vi "Add cell to table Header or Footer.vi"(4 "font":refnum<k24>, 5 "Close Cell ref (T)":bool=TRUE, 6 "Leading":T1=18.0, 7 "Aligment":string="JUSTIFY", 8 "error in (no error)":errorcluster, 9 "Cell format":T2={"Font"={"Name"="Helvetica", "Size"=12.0, "Color"=0, "Style"={"Bold"=FALSE, "Italic"=FALSE, "Underline"=FALSE, "Strikeout"=FALSE}}, "Align. and LS"={"Horizontal"=enum."LEFT", "Vertical"=enum."BOTTOM", "Line spacing"=enum."1.0"}, "Border"={"Show?"=FALSE, "Thickness (point)"=0.0, "Color"=0}}, 10 "String":string, 11 "PdfP Table":refnum<k24>) -> (0 "error out":errorcluster, 2 "Cell ref":refnum<k24>, 3 "PdfP Table duplicate":refnum<k24>)   [LabVIEW 2019]
doc: "Version 1.0\nDeveloped by Jean-Marc Simard\nCopyright © 2010, Exaprom Inc.\nAll rights reserved.\nLicense: BSD\n\nWith iTextSharp 4.1.6 (http://itextsharp.sourceforge.net)\nunder Mozilla Public License Version 1.1\n(http://www.mozilla.org/MPL/MPL-1.1.html)"
uses:
  C:/Program Files/National Instruments/LabVIEW 2019/user.lib/Exaprom PDF/DLL/itextsharp.dll
  DLL/itextsharp.dll
  <userlib>/Exaprom PDF/Controls/Cell Properties.ctl
  <userlib>/Exaprom PDF/Controls/Font Controls/Font cluster.ctl
  <userlib>/Exaprom PDF/Controls/Font Controls/Font size.ctl
  <userlib>/Exaprom PDF/Controls/Font Controls/Font color.ctl
  <userlib>/Exaprom PDF/Controls/Table Controls/Cell Vertical alignment.ctl
  <userlib>/Exaprom PDF/Controls/Text Controls/Line spacing.ctl
  <userlib>/Exaprom PDF/Controls/Image Controls/Image border.ctl
  <userlib>/Exaprom PDF/Controls/Text Controls/Texte alignement.ctl
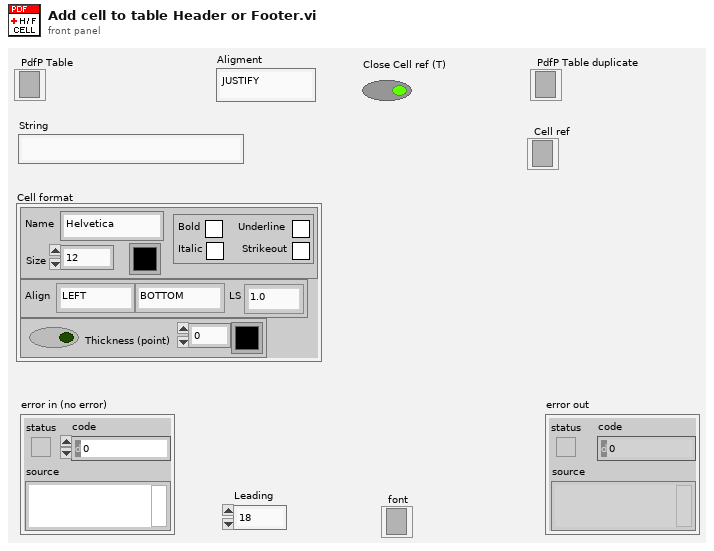
[diagram p1: front panel]
types:
  T1 = typedef "Font size.ctl" = sgl
  T2 = typedef "Cell Properties.ctl" = cluster{"Font":T3, "Align. and LS":cluster{"Horizontal":T5, "Vertical":T6, "Line spacing":T7}, "Border":T8}
  T3 = typedef "Font cluster.ctl" = cluster{"Name":string, "Size":T1, "Color":T4, "Style":cluster{"Bold":bool, "Italic":bool, "Underline":bool, "Strikeout":bool}}
  T4 = typedef "Font color.ctl" = u32
  T5 = typedef "Texte alignement.ctl" = enum16{"Select", "CENTER", "JUSTIFY", "LEFT", "RIGHT"}
  T6 = typedef "Cell Vertical alignment.ctl" = enum16{"TOP", "MIDDLE", "BOTTOM"}
  T7 = typedef "Line spacing.ctl" = enum16{"Select", "1.0", "1.5", "2.0"}
  T8 = typedef "Image border.ctl" = cluster{"Show?":bool, "Thickness (point)":sgl, "Color":u32}
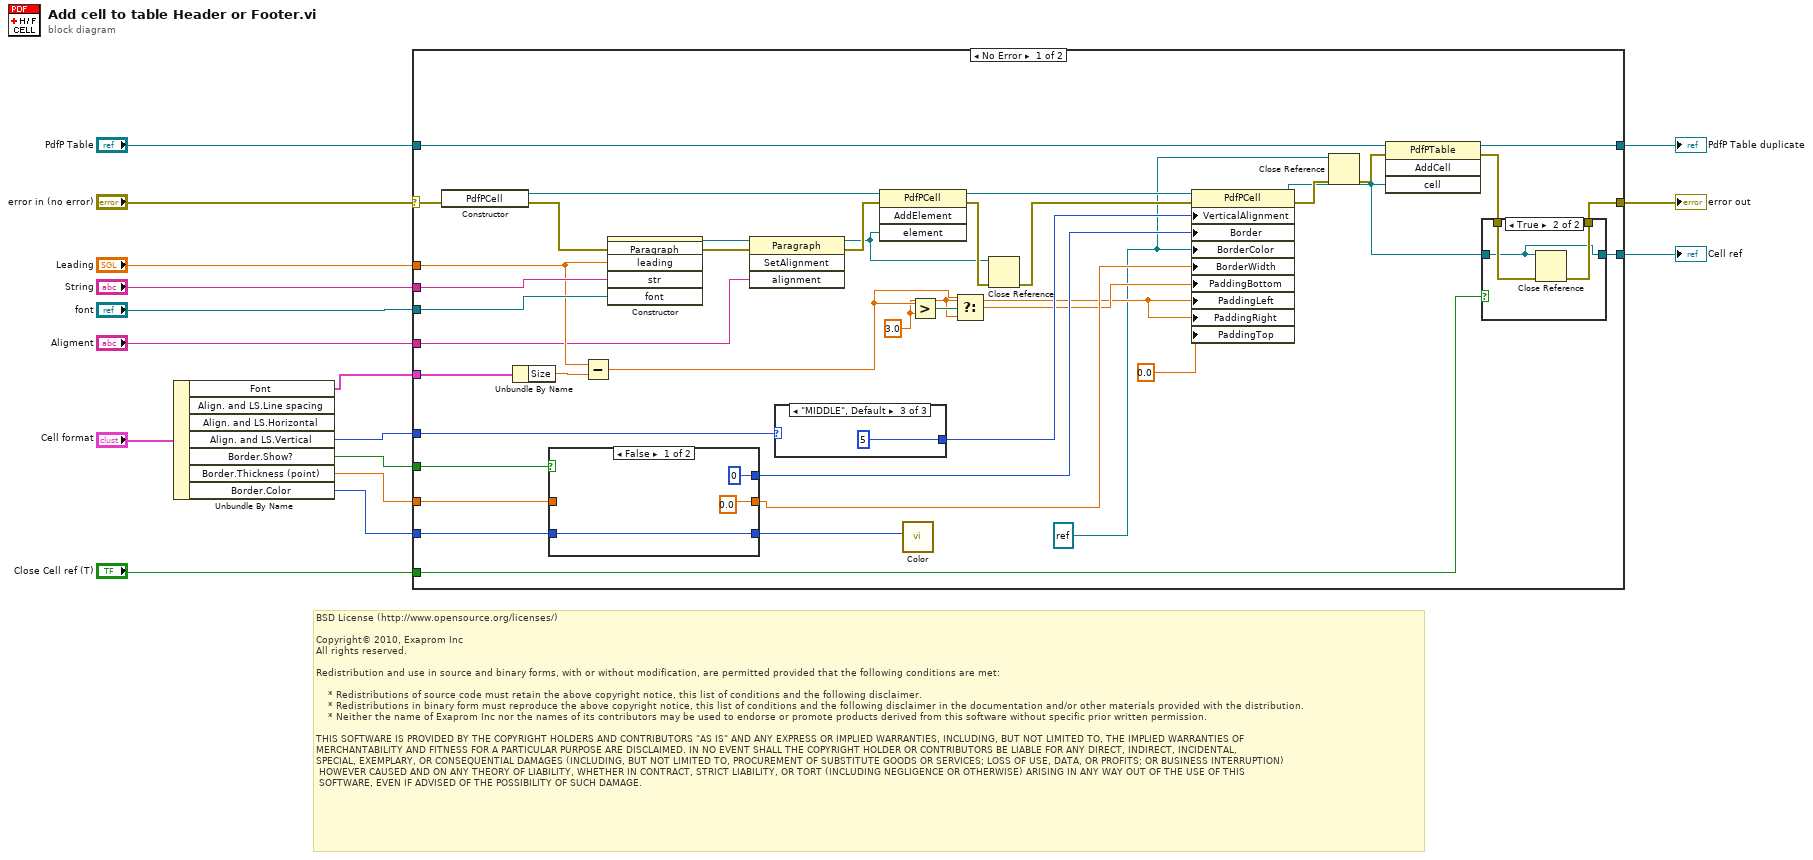
[diagram p0: block diagram]
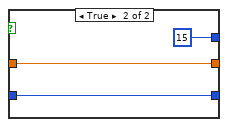
[diagram p3: hidden frame]
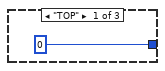
[diagram p4: hidden frame]
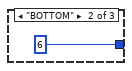
[diagram p5: hidden frame]
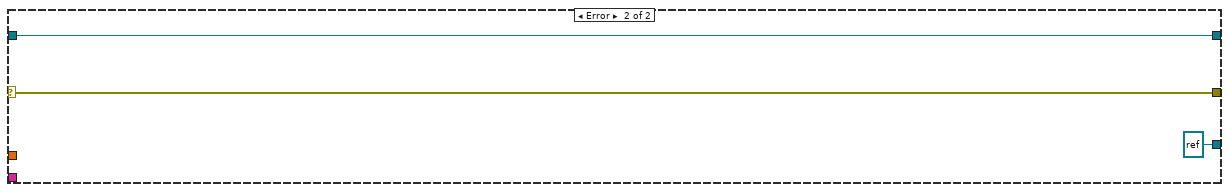
[diagram p6: hidden frame]
diagram:
  # "BSD License (http://www.opensource.org/licenses/)\n\nCopyright© 2010, Exaprom Inc\nAll rights reserved.\n\nRedistribution and use in source and binary forms, with or without modification, are permitted provided that the following conditions are met:\n\n    * Redistributions of source code must retain the above copyright notice, this list of conditions and the following disclaimer.\n    * Redistributions in binary form must reproduce the above copyright notice, this list of conditions and the following disclaimer in the documentation and/or other materials provided with the distribution.\n    * Neither the name of Exaprom Inc nor the names of its contributors may be used to endorse or promote products derived from this software without specific prior written permission.\n\nTHIS SOFTWARE IS PROVIDED BY THE COPYRIGHT HOLDERS AND CONTRIBUTORS \"AS IS\" AND ANY EXPRESS OR IMPLIED WARRANTIES, INCLUDING, BUT NOT LIMITED TO, THE IMPLIED WARRANTIES OF \nMERCHANTABILITY AND FITNESS FOR A PARTICULAR PURPOSE ARE DISCLAIMED. IN NO EVENT SHALL THE COPYRIGHT HOLDER OR CONTRIBUTORS BE LIABLE FOR ANY DIRECT, INDIRECT, INCIDENTAL,\nSPECIAL, EXEMPLARY, OR CONSEQUENTIAL DAMAGES (INCLUDING, BUT NOT LIMITED TO, PROCUREMENT OF SUBSTITUTE GOODS OR SERVICES; LOSS OF USE, DATA, OR PROFITS; OR BUSINESS INTERRUPTION)\n HOWEVER CAUSED AND ON ANY THEORY OF LIABILITY, WHETHER IN CONTRACT, STRICT LIABILITY, OR TORT (INCLUDING NEGLIGENCE OR OTHERWISE) ARISING IN ANY WAY OUT OF THE USE OF THIS\n SOFTWARE, EVEN IF ADVISED OF THE POSSIBILITY OF SUCH DAMAGE."
  n1 = Unbundle By Name("Cell format") -> ("Font"=w6:T3, "Align. and LS.Vertical"=w10:T6, "Border.Show?"=w9:bool, "Border.Thickness (point)"=w8:sgl, "Border.Color"=w7:u32)  [unwired: 2 out]
  n2 = case shown="No Error" "error in (no error)" {
    selector: "error in (no error)" -> [w51 w72]
    tunnel: [w35 w72] -> w15
    tunnel: [w18 w71] -> w14
    tunnel: "PdfP Table" -> [w50 w71]
    tunnel: w6 -> [w24 _]
    tunnel: "String" -> [w49 _]
    tunnel: w10 -> [w48 _]
    tunnel: w8 -> [w45 _]
    tunnel: w7 -> [w44 _]
    tunnel: w9 -> [w46 _]
    tunnel: "font" -> [w27 _]
    tunnel: "Leading" -> [w25 _]
    tunnel: "Aligment" -> [w23 _]
    tunnel: "Close Cell ref (T)" -> [w21 _]
    tunnel: [w20 refnum<k24> refnum ("new reference")] -> w1
    frame No Error {
      w19 = refnum<k24> refnum ("BorderColor")
      w28 = sgl 3.0 ("t")
      n3 = constructor class="PdfPCell"(error in=w51) -> (reference out=w55:refnum<k24>, error out=w22:errorcluster)  [unwired: 2 in, 1 out]
      n4 = Unbundle By Name(w24) -> ("Size"=w41:T1)
      n5 = case shown="False" w46 {
        tunnel: [sgl 0.0 ("BorderWidth") w65] -> w42
        tunnel: w45 -> [_ w65]
        tunnel: [w62 w64] -> w32
        tunnel: w44 -> [w62 w64]
        tunnel: [0 15] -> w43
        frame False {
        }
        frame True {
        }
      }
      n6 = Subtract(x=w25, y=w41) -> (x-y=w30:T1)
      n7 = constructor class="Paragraph"(error in=w22, "leading"=w25, "str"=w49, "font"=w27) -> (reference out=w54:refnum<k24>, error out=w26:errorcluster)  [unwired: 2 in, 4 out]
      n8 = invoke class="Paragraph" method="SetAlignment"(reference=w54, error in=w26, "alignment"=w23) -> (reference out=w38:refnum<k24>, error out=w53:errorcluster)  [unwired: 1 in, 2 out]
      n9 = case shown="\"MIDDLE\", Default" w48 {
        tunnel: [0 6 5] -> w47
        frame "TOP" {
        }
        frame "BOTTOM" {
        }
        frame "MIDDLE", Default {
        }
      }
      n10 = invoke class="PdfPCell" method="AddElement"(reference=w55, error in=w53, "element"=w38) -> (reference out=w52:refnum<k24>, error out=w39:errorcluster)  [unwired: 1 in, 2 out]
      n11 = call <userlib>:"Color.vi"("Color"=w32) -> ()  [unwired: 1 in, 10 out]
      n12 = Greater?(x=w30, y=w28) -> (0:w31:bool)
      n13 = Select(t=w30, s=w31, f=w28) -> (s? t:f=w29:T1)
      n14 = Close Reference(reference=w38, error in (no error)=w39) -> (error out=w33:errorcluster)
      n15 = property class="PdfPCell"(reference=w52, error in=w33, "VerticalAlignment"=w47, "Border"=w43, "BorderColor"=w19, "BorderWidth"=w42, "PaddingBottom"=w29, "PaddingLeft"=w28, "PaddingRight"=w28, "PaddingTop"=sgl 0.0) -> (reference out=w34:refnum<k24>, error out=w37:errorcluster)
      n16 = Close Reference(reference=w19, error in (no error)=w37) -> (error out=w36:errorcluster)
      n17 = invoke class="PdfPTable" method="AddCell"(reference=w50, error in=w36, "cell"=w34) -> (reference out=w18:refnum<k24>, error out=w17:errorcluster)  [unwired: 1 in, 2 out]
      n18 = case shown="True" w21 {
        tunnel: w17 -> [w57 w60]
        tunnel: [w57 w59] -> w35
        tunnel: w34 -> [w56 w58]
        tunnel: [w56 w58] -> w20
        frame False {
        }
        frame True {
          n19 = Close Reference(reference=w58, error in (no error)=w60) -> (error out=w59:errorcluster)
        }
      }
    }
    frame Error {
    }
  }
  "error out" <- w15
  "PdfP Table duplicate" <- w14
  "Cell ref" <- w1
